vi "FTW-TransferClient-UploadBegin.vi"(0 "Transfer Client":refnum<class "FTW-TransferClient-dotNET.lvclass">, 5 "Local Filepath":path, 7 "Remote Relative Filepath":string, 11 "error in":errorcluster) -> (4 "Transfer Client out":refnum<class "FTW-TransferClient-dotNET.lvclass">, 6 "Upload Events":refnum<event-registration>, 15 "error out":errorcluster)   [LabVIEW 2013, in "FTW-TransferClient-dotNET.lvclass"]
uses:
  FTW-TransferClient-dotNET.lvclass
  FTW-TransferClient-TransferProgress.ctl
  FTW-TransferClient-TransferStatus.ctl
  FTW-TransferClient-dotNET.lvclass/FTW-TransferClient-dotNET.ctl
  FTW-TransferClient.lvclass
panel:
  # "Inputs"
  # "Outputs"
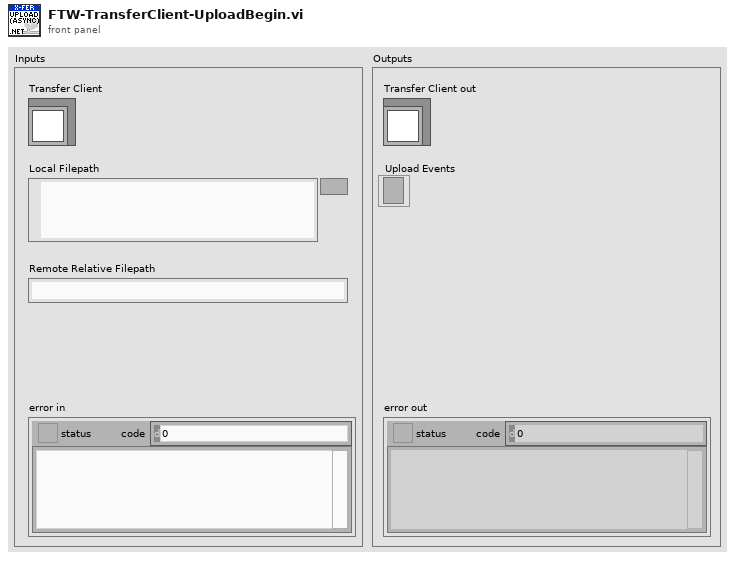
[diagram p1: front panel]
types:
  T1 = cluster{"Transfer Complete":refnum<user-event>, "Transfer Begin Timestamp":u32, "AbsoluteURI":string, "Local Filepath":path}
  T2 = cluster{"Transfer Progress":refnum<user-event>, "Transfer Begin Timestamp":u32, "AbsoluteURI":string, "Local Filepath":path}
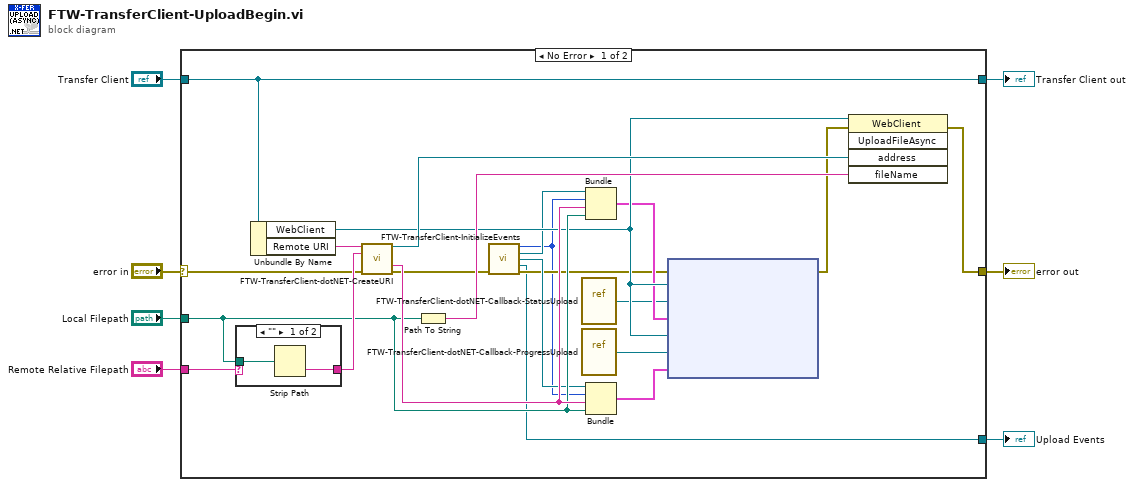
[diagram p0: block diagram]
diagram:
  n1 = case shown="No Error" "error in" {
    selector: "error in" -> [w21 w33]
    tunnel: "Transfer Client" -> [w25 w34]
    tunnel: [w20 w33] -> w6
    tunnel: [w25 w34] -> w7
    tunnel: "Local Filepath" -> [w22 _]
    tunnel: "Remote Relative Filepath" -> [w24 _]
    tunnel: [w9 _] -> w5
    frame No Error {
      n2 = case shown="\"\"" w24 {
        selector: w24 -> [_ w32]
        tunnel: w22 -> [w31 _]
        tunnel: [w30 w32] -> w23
        frame "" {
          n3 = Strip Path(path=w31) -> (name=w30:string)  [unwired: 1 out]
        }
        frame Default {
        }
      }
      n4 = Unbundle By Name(w25) -> ("WebClient"=w17:refnum<k24>, "Remote URI"=w28:string)
      n5 = call "FTW-TransferClient-dotNET-CreateURI.vi"("URI"=w28, "Relative URI"=w23, "error in"=w21) -> ("URI ref"=w27:refnum<k24>, "AbsoluteURI"=w26:string, "error out"=w11:errorcluster)  [unwired: 7 in, 3 out]
      n6 = Path To String(path=w22) -> (string=w29:string)
      n7 = call "FTW-TransferClient-InitializeEvents.vi"("error in"=w11) -> ("Transfer Begin Timestamp"=w8:u32, "Transfer Complete"=w12:refnum<user-event>, "Transfer Progress"=w13:refnum<user-event>, "Transfer Events"=w9:refnum<event-registration>, "error out"=w10:errorcluster)  [unwired: 10 in]
      n8 = vi-ref "FTW-TransferClient-dotNET-Callback-StatusUpload.vi"() -> ("vi reference"=w15:refnum<vi>)
      n9 = vi-ref "FTW-TransferClient-dotNET-Callback-ProgressUpload.vi"() -> ("vi reference"=w14:refnum<vi>)
      n10 = Bundle("Transfer Complete"=w12, "Transfer Begin Timestamp"=w8, "AbsoluteURI"=w26, "Local Filepath"=w22) -> (w16:T1)  [unwired: 1 in]
      n11 = Bundle("Transfer Progress"=w13, "Transfer Begin Timestamp"=w8, "AbsoluteURI"=w26, "Local Filepath"=w22) -> (w19:T2)  [unwired: 1 in]
      n12 = node(w10, w17, w15, w16, w17, w14, w19) -> (w18:errorcluster)  [unwired: 1 in, 1 out]
      n13 = invoke class="WebClient" method="UploadFileAsync"(reference=w17, error in=w18, "address"=w27, "fileName"=w29) -> (error out=w20:errorcluster)  [unwired: 1 in, 4 out]
    }
    frame Error {
    }
  }
  "error out" <- w6
  "Transfer Client out" <- w7
  "Upload Events" <- w5
